vi "config.vi"(8 "error in (no error)":errorcluster, 10 "Configuration":T1={"Config Dir"=path "/home/ttsai/Documents/stash/ts_tcs_ofc/configData", "Bending Mode Files"={"M1M3 Subsystem"={"Mirror"="M1M3", "Actuatro Force File"="M1M3_1um_156_force.txt"}, "M2 Subsystem"={"Mirror"="M2", "Actuatro Force File"="M2_1um_force.DAT"}, "Num of Bending Mode"=20}, "Rot Mirror FEA File Name"="rotMat_Bo_to_Chris_FEA_DOF.txt"}, 11 "BendModeToForce in":refnum<class "BendModeToForce.lvclass">) -> (0 "error out":errorcluster, 3 "BendModeToForce out":refnum<class "BendModeToForce.lvclass">)   [LabVIEW 2016, in "BendModeToForce.lvclass"]
doc: "Do the configuration of bending mode to forces (BMTF)."
uses:
  BendModeToForce.lvclass
  BendModeToForce.lvclass/BendModeToForce.ctl
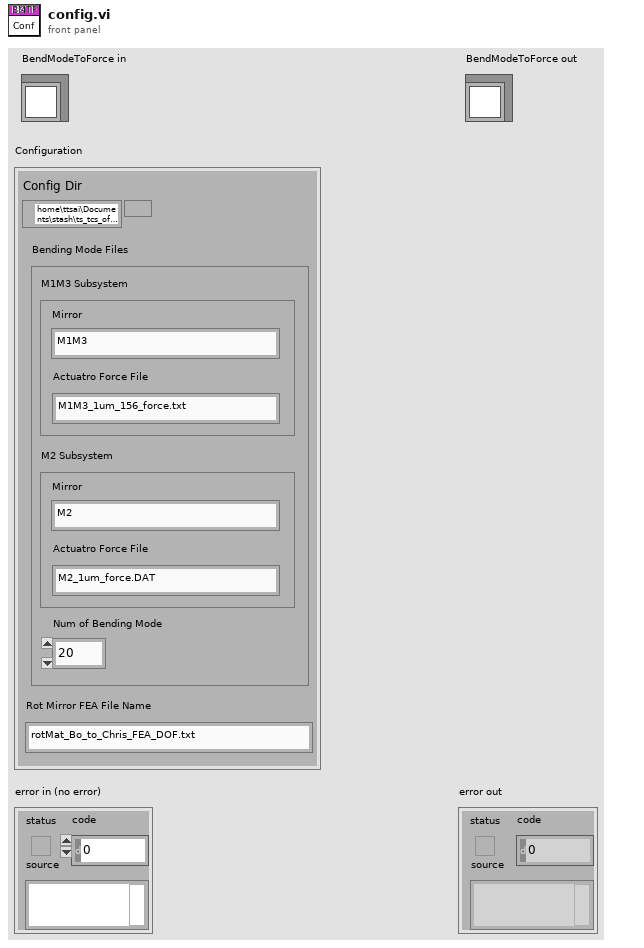
[diagram p1: front panel]
types:
  T1 = cluster{"Config Dir":path, "Bending Mode Files":cluster{"M1M3 Subsystem":cluster{"Mirror":string, "Actuatro Force File":string}, "M2 Subsystem":cluster{"Mirror":string, "Actuatro Force File":string}, "Num of Bending Mode":i32}, "Rot Mirror FEA File Name":string}
  T2 = cluster{"Mirror":string, "Actuatro Force File":string}
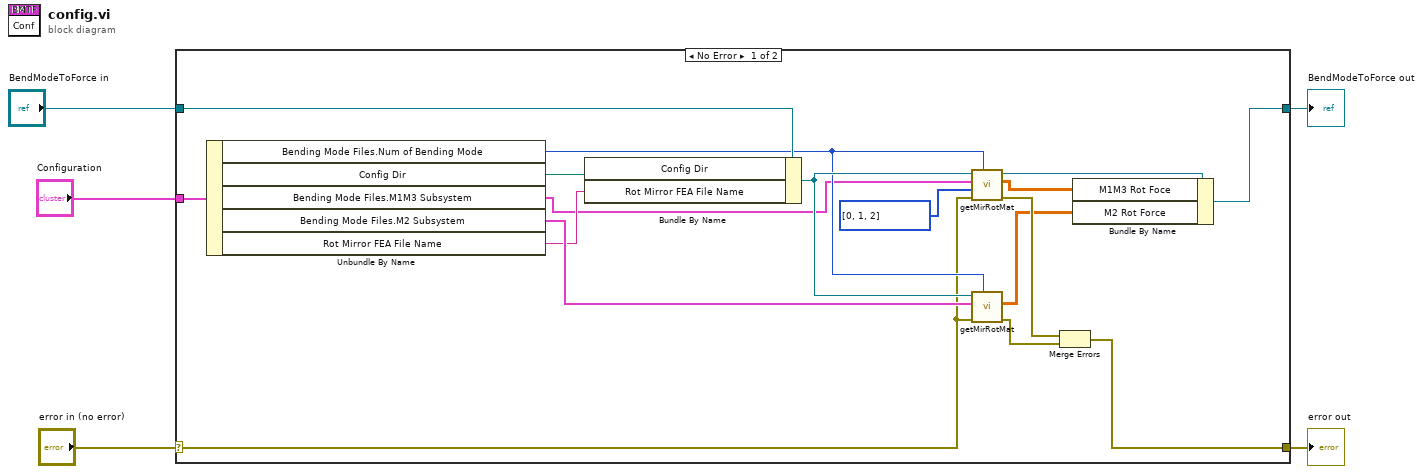
[diagram p0: block diagram]
diagram:
  n1 = case shown="No Error" "error in (no error)" {
    selector: "error in (no error)" -> [w15 w24]
    tunnel: [w12 w24] -> w4
    tunnel: [w8 w23] -> w2
    tunnel: "BendModeToForce in" -> [w22 w23]
    tunnel: "Configuration" -> [w21 _]
    frame No Error {
      n2 = Unbundle By Name(w21) -> ("Bending Mode Files.Num of Bending Mode"=w16:i32, "Config Dir"=w19:path, "Bending Mode Files.M1M3 Subsystem"=w6:T2, "Bending Mode Files.M2 Subsystem"=w18:T2, "Rot Mirror FEA File Name"=w7:string)
      n3 = Bundle By Name(cluster=w22, "Config Dir"=w19, "Rot Mirror FEA File Name"=w7) -> (w20:refnum<class "BendModeToForce.lvclass">)
      n4 = call "getMirRotMat.vi"("Num of Bending Mode"=w16, "error in (no error)"=w15, "Skip Col Idx"=i32[] [0, 1, 2], "Mirror Subsystem"=w6, "BendModeToForce in"=w20) -> ("error out"=w14:errorcluster, "Rotation Matrix"=w10:dbl[][], "BendModeToForce out"=w11:refnum<class "BendModeToForce.lvclass">)  [unwired: 4 in]
      n5 = call "getMirRotMat.vi"("Num of Bending Mode"=w16, "error in (no error)"=w15, "Mirror Subsystem"=w18, "BendModeToForce in"=w20) -> ("error out"=w13:errorcluster, "Rotation Matrix"=w9:dbl[][])  [unwired: 5 in, 1 out]
      n6 = Merge Errors(w14, w13) -> (w12:errorcluster)
      n7 = Bundle By Name(cluster=w11, "M1M3 Rot Foce"=w10, "M2 Rot Force"=w9) -> (w8:refnum<class "BendModeToForce.lvclass">)
    }
    frame Error {
    }
  }
  "error out" <- w4
  "BendModeToForce out" <- w2
